vi "Disable Measurements.vi"(0 "Register Buses":T1[](array[typedef]), 11 "error in":errorcluster) -> (4 "Register Buses (out)":T1[](array[typedef]), 15 "error out":errorcluster)   [LabVIEW 2014, in "ni579x Synchronization v2 Host.lvlib"]
doc: "Turn off the measurement circuits on the FPGA."
uses:
  <instrlib>/ni579x/Synchronization/v2/Host/ni579x Synchronization v2 Host.lvlib
  <instrlib>/_niInstr/Register Bus/v0/Host/Public/Register Bus Session.ctl
  <instrlib>/_niInstr/Register Bus/v0/Host/Private/Session Data.ctl
  <instrlib>/ni579x/Synchronization/v2/Shared/ni579x Synchronization Register Addresses.ctl
  <instrlib>/ni579x/Config/v2/Shared/Types/ni579x Register Bus Subsystem ID.ctl
  <instrlib>/_niInstr/Register Bus/v0/Host/Public/Register Write.ctl
  <instrlib>/ni579x/Config/v2/Shared/ni579x Config v2 Shared.lvlib
  <instrlib>/_niInstr/Register Bus/v0/Host/niInstr Register Bus v0 Host.lvlib
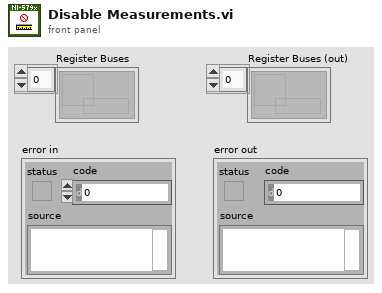
[diagram p1: front panel]
types:
  T1 = typedef "niInstr Register Bus v0 Host.lvlib/Register Bus Session.ctl" = refnum<queue>
  T2 = typedef "niInstr Register Bus v0 Host.lvlib/Register Write.ctl" = cluster{"subsystem":u8, "address":u16, "data":u32}
  T3 = typedef "ni579x Config v2 Shared.lvlib/ni579x Register Bus Subsystem ID.ctl" = u8
  T4 = typedef "ni579x Synchronization Register Addresses.ctl" = enum16{"Signature", "Current Version", "Oldest Compatible Version", "Scratch Register", "sync.master", "sync.meas.enable", "sync.meas.ready", "sync.meas.arm", "sync.meas.valid", "sync.meas.value", "sync.cptr.adjust", "sync.cptr.period", "sync.meas.oversample factor"}
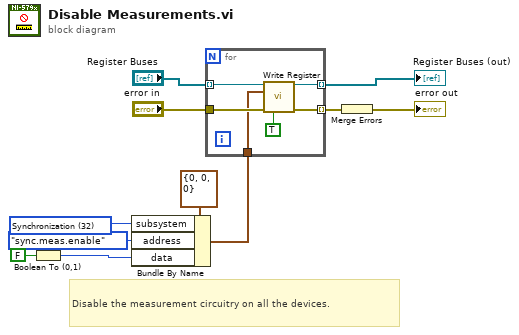
[diagram p0: block diagram]
diagram:
  w9 = T3 32 items=["FAM Register Operation"=0, "User Command"=16, "Synchronization"=32] ("Subsystem ID")
  # "Disable the measurement circuitry on all the devices."
  n1 = Boolean To (0,1)(Boolean=FALSE ("sync.Master")) -> (0, 1=w11:i16)
  n2 = Bundle By Name(cluster=T2 {"subsystem"=0, "address"=0, "data"=0} ("register write"), "subsystem"=w9, "address"=ni579x_Synchronization_Register_Addresses."sync.meas.enable" ("Synchronization Registers"), "data"=w11) -> (w7:T2)
  n3 = for {
    tunnel: "Register Buses" -> [w17] mode=indexing
    tunnel: w7 -> [w15]
    tunnel: [w13] -> w2 mode=indexing
    tunnel: "error in" -> [w16]
    tunnel: [w12] -> w4 mode=indexing
    n4 = call <instrlib>:"Write Register.vi"("session in"=w17, "register write"=w15, "error in"=w16, "wait until committed"=TRUE) -> ("session out"=w13:T1, "error out"=w12:errorcluster)  [unwired: 10 in]
  }
  "Register Buses (out)" <- w2
  n5 = Merge Errors(w4) -> (→"error out":errorcluster)
